vi "Get Gyro Data.vi"(0 "LINX Resource In":T2, 1 "I2C Channel":u8, 11 "error in (no error)":errorcluster) -> (4 "LINX Resource Out":T2, 6 "Gyro Data":T1, 15 "error out":errorcluster)   [LabVIEW 2014, in "LMH-LINX.lvlib" / "ITG3200.lvlib"]
uses:
  <vilib>/MakerHub/LINX/Public/Sensors/Gyroscopes/ITG3200/ITG3200.lvlib
  <vilib>/MakerHub/LINX/Private/Type Defs/LINX Ref.ctl
  <vilib>/MakerHub/LINX/Private/Type Defs/Platform.ctl
  <vilib>/MakerHub/LINX/Private/Type Defs/Interface.ctl
  <vilib>/MakerHub/LINX/Private/Device/Type Defs/LINX Device Config.ctl
  <vilib>/MakerHub/LINX/Private/Device/Type Defs/TCP Config.ctl
  <vilib>/MakerHub/LINX/Private/Device/Type Defs/Channels.ctl
  <vilib>/MakerHub/LINX/Public/Sensors/Gyroscopes/ITG3200/Controls/Gyro_Data.ctl
  <vilib>/MakerHub/LINX/Private/Local IO/LinxI2cWrite.vi
  <vilib>/MakerHub/LINX/Public/Utilities/Check Channel.vi
  <vilib>/MakerHub/LINX/Private/Utilties/Generate Error.vi
  <vilib>/MakerHub/LINX/LMH-LINX.lvlib
  <vilib>/MakerHub/Toolbox/LMH-Toolbox.lvlib
  <vilib>/MakerHub/LINX/Private/Device/Device.lvlib
panel:
  # "INPUTS"
  # "OUTPUTS"
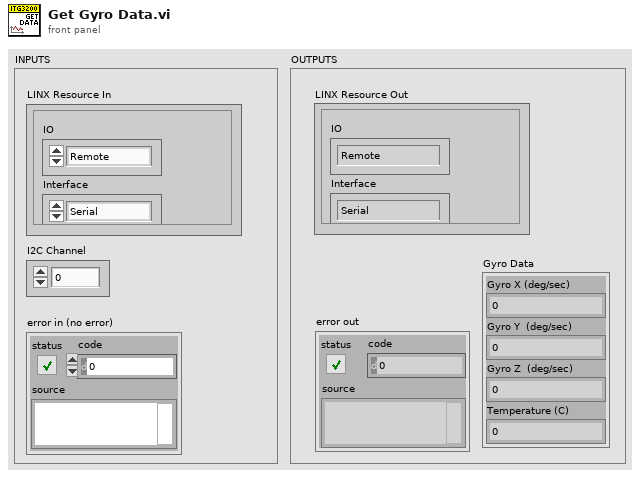
[diagram p1: front panel]
types:
  T1 = typedef "Gyro_Data.ctl" = cluster{"Gyro X (deg/sec)":i32, "Gyro Y  (deg/sec)":i32, "Gyro Z  (deg/sec)":i32, "Temperature (C)":i32}
  T2 = typedef "LMH-LINX.lvlib/LINX Ref.ctl" = cluster{"IO":T3, "Interface":T4, "LINX Device Config":T5}
  T3 = typedef "LMH-LINX.lvlib/Platform.ctl" = enum16{"Remote", "Local"}
  T4 = typedef "LMH-LINX.lvlib/Interface.ctl" = enum16{"Serial", "TCP"}
  T5 = typedef "LMH-LINX.lvlib/Device.lvlib/LINX Device Config.ctl" = cluster{"Interface":T4, "COM Port":refnum<visa-resource-name>, "TCP Configuration":T6, "Device Family":u8, "Device ID":u8, "Device Name":string, "TCP Ref":refnum<k5>, "Channels":T7}
  T6 = typedef "LMH-LINX.lvlib/Device.lvlib/TCP Config.ctl" = cluster{"IP Address":string, "Port":u16}
  T7 = typedef "LMH-LINX.lvlib/Channels.ctl" = cluster{"DI":u8[], "DO":u8[], "AI":u8[], "AO":u8[], "PWM":u8[], "QE":u8[], "UART":u8[], "I2C 2":u8[], "SPI":u8[], "CAN":u8[], "Servo":u8[], "AI Ref (V)":dbl, "AI Resolution (Bits)":u8, "AO Ref (V)":dbl, "AO Resolution (Bits)":u8}
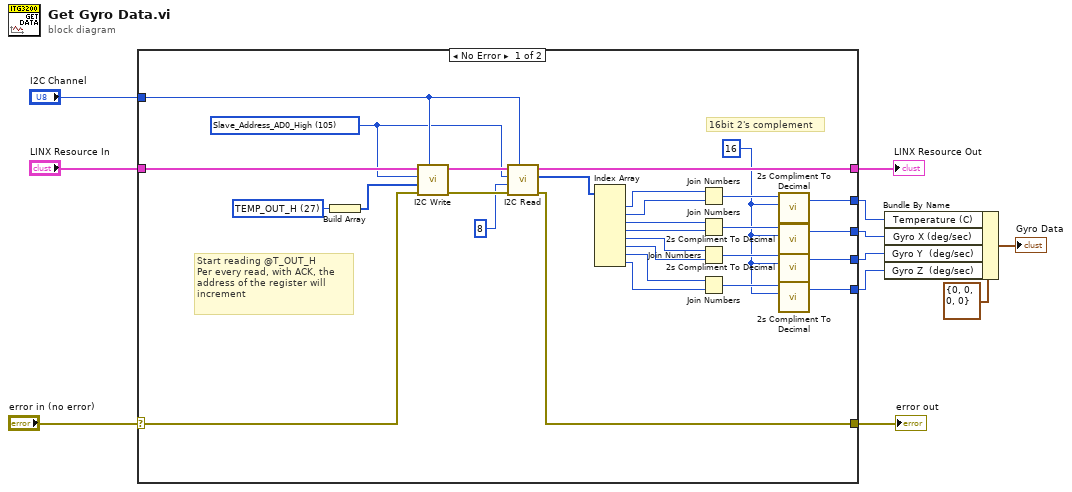
[diagram p0: block diagram]
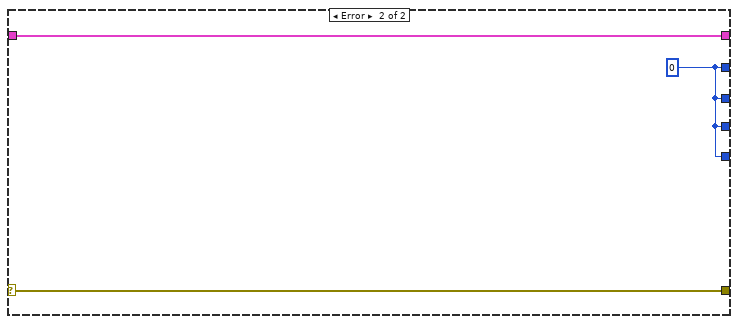
[diagram p2: hidden frame]
diagram:
  n1 = case shown="No Error" "error in (no error)" {
    selector: "error in (no error)" -> [w39 w43]
    tunnel: [w38 w43] -> w10
    tunnel: "LINX Resource In" -> [w40 w42]
    tunnel: "I2C Channel" -> [w36 _]
    tunnel: [w37 w42] -> w7
    tunnel: [w15 w41] -> w5
    tunnel: [w14 w41] -> w4
    tunnel: [w13 w41] -> w3
    tunnel: [w12 w41] -> w2
    frame No Error {
      w16 = 16
      w35 = u8 27 items=["WHO_AM_I"=0, "SMPLRT_DIV"=21, "DLPF_FS"=22, "INT_CFG"=23, "INT_STATUS"=26, "TEMP_OUT_H"=27, "TEMP_OUT_L"=28, "GYRO_XOUT_H"=29, "GYRO_XOUT_L"=30, "GYRO_YOUT_H"=31, "GYRO_YOUT_L"=32, "GYRO_ZOUT_H"=33, "GYRO_ZOUT_L"=34, "PWR_MGM"=62] ("Register Map")
      w31 = u8 105 items=["Slave_Address_AD0_Low"=104, "Slave_Address_AD0_High"=105] ("Slave Addresses")
      # "16bit 2's complement"
      # "Start reading @T_OUT_H\nPer every read, with ACK, the \naddress of the register will\nincrement"
      n2 = Build Array(w35) -> (w34:u8[])
      n3 = call <vilib>:"I2C Write.vi"("I2C Channel"=w36, "Error In"=w39, "Data"=w34, "I2C Slave Address (0)"=w31, "LINX Resource"=w40) -> ("Error Out"=w32:errorcluster, "LINX Resource"=w33:T2)  [unwired: 5 in]
      n4 = call <vilib>:"I2C Read.vi"("I2C Channel"=w36, "Error In"=w32, "Bytes To Read"=u8 8, "I2C Slave Address (0)"=w31, "LINX Resource"=w33) -> ("Error Out"=w38:errorcluster, "Data"=w29:u8[], "LINX Resource"=w37:T2)  [unwired: 4 in]
      n5 = Index Array(array=w29) -> (element #1=w28:u8, element #2=w27:u8, element #3=w26:u8, element #4=w25:u8, element #5=w24:u8, element #6=w23:u8, element #7=w22:u8, element #8=w21:u8)  [unwired: 8 in]
      n6 = Join Numbers(hi=w28, lo=w27) -> ((hi.lo)=w20:u16)
      n7 = Join Numbers(hi=w26, lo=w25) -> ((hi.lo)=w19:u16)
      n8 = Join Numbers(hi=w24, lo=w23) -> ((hi.lo)=w18:u16)
      n9 = Join Numbers(hi=w22, lo=w21) -> ((hi.lo)=w17:u16)
      n10 = call <vilib>:"2s Compliment To Decimal.vi"("Bit Width (8)"=w16, "2s Comp Number"=w20) -> ("Decimal Number"=w15:i32)  [unwired: 3 in]
      n11 = call <vilib>:"2s Compliment To Decimal.vi"("Bit Width (8)"=w16, "2s Comp Number"=w19) -> ("Decimal Number"=w14:i32)  [unwired: 3 in]
      n12 = call <vilib>:"2s Compliment To Decimal.vi"("Bit Width (8)"=w16, "2s Comp Number"=w18) -> ("Decimal Number"=w13:i32)  [unwired: 3 in]
      n13 = call <vilib>:"2s Compliment To Decimal.vi"("Bit Width (8)"=w16, "2s Comp Number"=w17) -> ("Decimal Number"=w12:i32)  [unwired: 3 in]
    }
    frame Error {
      w41 = 0 ("Decimal Number")
    }
  }
  "error out" <- w10
  "LINX Resource Out" <- w7
  n14 = Bundle By Name(cluster=T1 {"Gyro X (deg/sec)"=0, "Gyro Y  (deg/sec)"=0, "Gyro Z  (deg/sec)"=0, "Temperature (C)"=0} ("Gyro Data"), "Temperature (C)"=w5, "Gyro X (deg/sec)"=w4, "Gyro Y  (deg/sec)"=w3, "Gyro Z  (deg/sec)"=w2) -> (→"Gyro Data":T1)
